vi "Init Actor Core.vi"(8 "error in (no error)":errorcluster, 11 "Measure Object in":refnum<class "TCP Communications.lvclass">) -> (0 "error out":errorcluster, 3 "Measure Object out":refnum<class "TCP Communications.lvclass">)   [LabVIEW 2018, in "TCP Communications.lvclass"]
uses:
  TCP Communications.lvclass
  Communications/Communications.lvclass
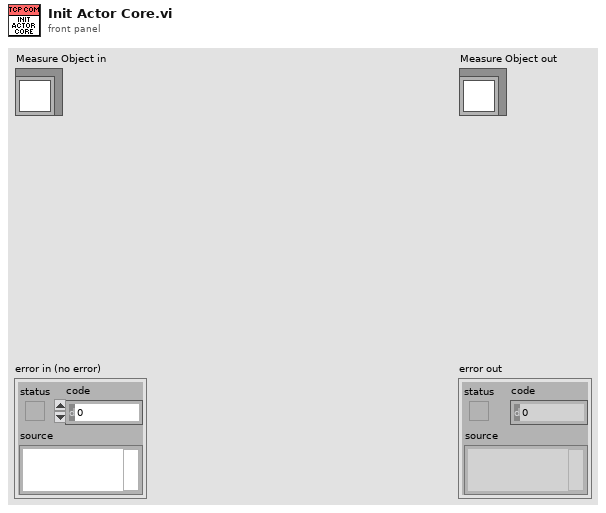
[diagram p1: front panel]
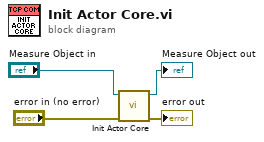
[diagram p0: block diagram]
diagram:
  n1 = call-parent "Init Actor Core.vi"("error in (no error)"="error in (no error)", "Measure Object in"="Measure Object in") -> ("error out"=→"error out":errorcluster, "Measure Object out"=→"Measure Object out":refnum<class "TCP Communications.lvclass">)  [unwired: 8 in]
